vi "create color value.vi"(2 "color":T1={"color array"=[0, 16711680, 16448250, 16448250, 16776960, 16711680, 16448250, 16448250], "num of colors"=3, "max"=340.0, "min"=20.0} {"min" step=0.01 format="%_2f"; "max" step=0.1 format="%_3f"}, 3 "input value":dbl) -> (1 "color value":u32(colorbox))   [LabVIEW 2024]
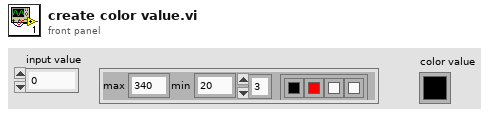
[diagram p1: front panel]
types:
  T1 = cluster{"color array":u32[], "num of colors":i32, "max":dbl, "min":dbl}
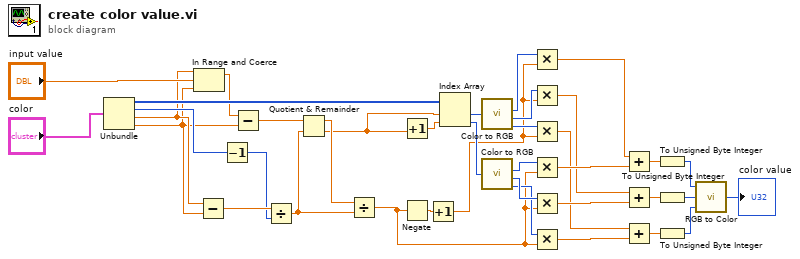
[diagram p0: block diagram]
diagram:
  n1 = Unbundle("color") -> ("color array"=w29:u32[], "num of colors"=w38:i32, "max"=w3:dbl, "min"=w2:dbl)
  n2 = In Range and Coerce(upper limit=w3, x="input value", lower limit=w2) -> (coerced(x)=w1:dbl)  [unwired: 1 out]
  n3 = Subtract(x=w3, y=w2) -> (x-y=w36:dbl)
  n4 = Decrement(x=w38) -> (x-1=w31:i32)
  n5 = Subtract(x=w1, y=w2) -> (x-y=w35:dbl)
  n6 = Divide(x=w36, y=w31) -> (x/y=w33:dbl)
  n7 = Quotient & Remainder(x=w35, y=w33) -> (x-y*floor(x/y)=w34:dbl, floor(x/y)=w32:dbl)
  n8 = Divide(x=w34, y=w33) -> (x/y=w5:dbl)
  n9 = Increment(x=w32) -> (x+1=w30:dbl)
  n10 = Negate(x=w5) -> (-x=w28:dbl)
  n11 = Increment(x=w28) -> (x+1=w6:dbl)
  n12 = Index Array(array=w29, index #1=w32, index #2=w30) -> (element #1=w14:u32, element #2=w13:u32)
  n13 = call <vilib>:"Color to RGB.vi"("Color"=w14) -> ("R"=w12:u8, "G"=w11:u8, "B"=w10:u8)  [unwired: 1 out]
  n14 = call <vilib>:"Color to RGB.vi"("Color"=w13) -> ("R"=w9:u8, "G"=w8:u8, "B"=w7:u8)  [unwired: 1 out]
  n15 = Multiply(x=w12, y=w6) -> (x*y=w27:dbl)
  n16 = Multiply(x=w11, y=w6) -> (x*y=w25:dbl)
  n17 = Multiply(x=w10, y=w6) -> (x*y=w23:dbl)
  n18 = Multiply(x=w9, y=w5) -> (x*y=w26:dbl)
  n19 = Multiply(x=w8, y=w5) -> (x*y=w24:dbl)
  n20 = Multiply(x=w7, y=w5) -> (x*y=w22:dbl)
  n21 = Add(x=w27, y=w26) -> (x+y=w18:dbl)
  n22 = Add(x=w25, y=w24) -> (x+y=w17:dbl)
  n23 = Add(x=w23, y=w22) -> (x+y=w16:dbl)
  n24 = To Unsigned Byte Integer(number=w18) -> (unsigned 8bit integer=w19:u8)
  n25 = To Unsigned Byte Integer(number=w17) -> (unsigned 8bit integer=w20:u8)
  n26 = To Unsigned Byte Integer(number=w16) -> (unsigned 8bit integer=w21:u8)
  n27 = call <vilib>:"RGB to Color.vi"("B"=w21, "G"=w20, "R"=w19) -> ("Color"=→"color value":u32)
